vi "HB_RefNumRegistrySet.vi"(0 "HBDevRef":T1, 5 "refnum name":string, 11 "error in (no error)":errorcluster) -> (4 "HBDevRef":T1, 15 "error out":errorcluster)   [LabVIEW 2016]
uses:
  <vilib>/Rock Robotics/WPI/SerialPort/WPI_SerialPortRef.ctl
  <vilib>/Rock Robotics/WPI/Utilities/Refnum Registry Operation.ctl
panel:
  in  "Test Mode Only":bool
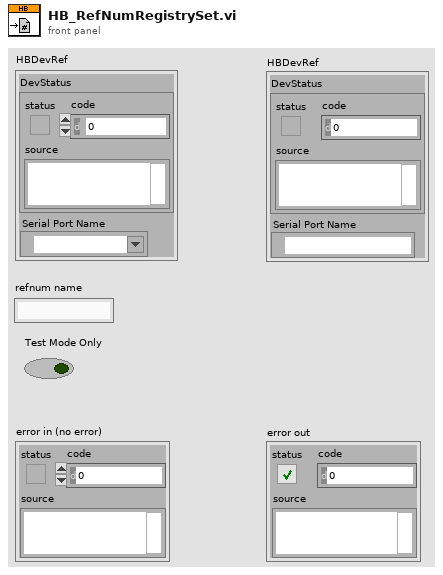
[diagram p1: front panel]
types:
  T1 = typedef "WPI_SerialPortRef.ctl" = cluster{"DevStatus":errorcluster, "Serial Port Name":refnum<visa-resource-name>}
  T2 = typedef "Refnum Registry Operation.ctl" = enum16{"set", "get", "delete", "get all names", "read name"}
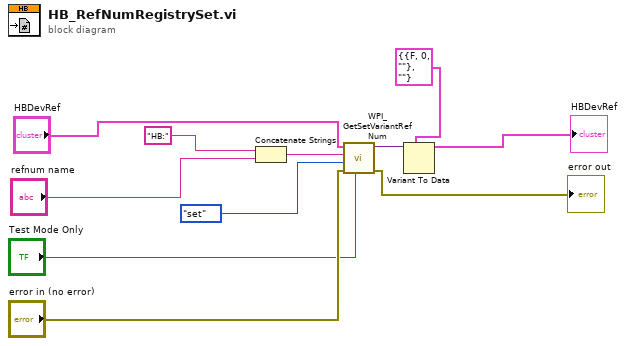
[diagram p0: block diagram]
diagram:
  n1 = Concatenate Strings("HB:", "refnum name") -> (w11:string)
  n2 = call <vilib>:"WPI_GetSetVariantRefNum.vi"("Test Mode Only"="Test Mode Only", "error in (no error)"="error in (no error)", "Operation"=Refnum_Registry_Operation."set" ("menu"), "refnum name"=w11, "DevRef"="HBDevRef") -> ("error out"=→"error out":errorcluster, "DevRef"=w3:variant)  [unwired: 4 in, 1 out]
  n3 = Variant To Data(type=T1 {"DevStatus"={"status"=FALSE, "code"=0, "source"=""}, "Serial Port Name"=""} ("HBDevRef 2"), Variant=w3) -> (data=→"HBDevRef":T1)  [unwired: 1 in, 1 out]
